vi "image to matrix.vi"(10 "matrixSize":i32, 11 "Image Path":path) -> (3 "matrix out 2D":dbl[][](array[numeric]))   [LabVIEW 2012, in "LightPipes.lvlib"]
doc: "__declspec(dllexport) void image_to_matrix(const char *path, int matrixSize, double matrix[]);"
uses:
  LightPipes.lvlib
  Lightpipes.dll
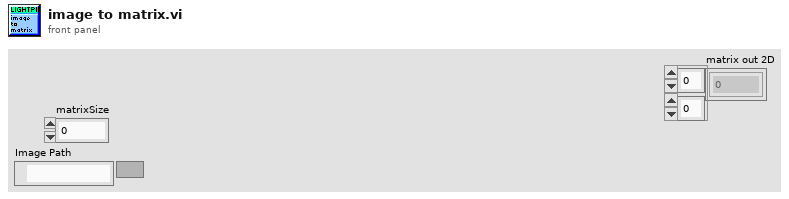
[diagram p1: front panel]
types:
  T1 = enum16{"open", "replace", "create", "open or create", "replace or create", "replace or create with confirmation"}
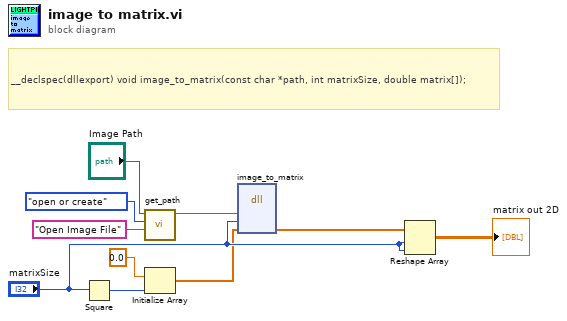
[diagram p0: block diagram]
diagram:
  # "__declspec(dllexport) void image_to_matrix(const char *path, int matrixSize, double matrix[]);"
  n1 = Square(x="matrixSize") -> (x^2=w10:i32)
  n2 = call "get_path.vi"("Message Prompt"="Open Image File", "operation (default: open/create)"=T1."open or create", "Path In"="Image Path") -> ("Path out"=w1:string)  [unwired: 8 in]
  n3 = Initialize Array "Initialize Array"(0.0 ("element"), w10) -> (w6:dbl[])
  n4 = dll-call lib="C:/Users/Tri/Documents/Gerchberg/Lightpipes.*" fn="image_to_matrix"("path"=w1, "matrixSize"="matrixSize", "matrix"=w6) -> ("matrix"=w5:dbl[])  [unwired: 6 in, 2 out]
  n5 = Reshape Array "Reshape Array"(w5, "matrixSize", "matrixSize") -> (→"matrix out 2D":dbl[][])
